vi "CheckForSaturation.vi"(8 "Replace Sat with X?":dbl=0.1 format="%#_13g", 9 "Processed Data":dbl[][](array[numeric]), 10 "Original Data In":dbl[][](array[numeric]), 11 "Bit Depth":i32=8) -> (3 "Data with Saturation":dbl[][](array[numeric]))   [LabVIEW 2022 SP3]
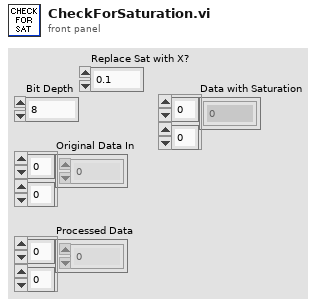
[diagram p1: front panel]
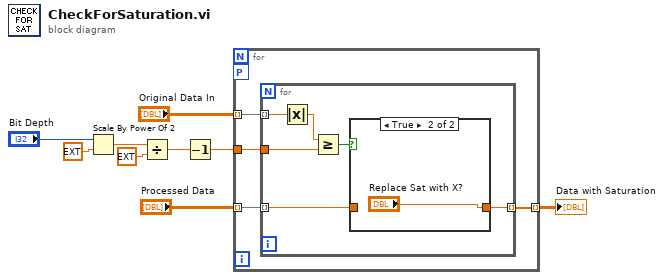
[diagram p0: block diagram]
diagram:
  n1 = Scale By Power Of 2(n="Bit Depth", x=ext 1.0) -> (x*2^n=w5:ext)
  n2 = Divide(x=w5, y=ext 2.0) -> (x/y=w7:ext)
  n3 = Decrement(x=w7) -> (x-1=w9:ext)
  n4 = for {
    tunnel: [w13] -> w2 mode=indexing
    tunnel: "Processed Data" -> [w12] mode=indexing
    workers-P: _ -> [_]
    tunnel: "Original Data In" -> [w11] mode=indexing
    tunnel: w9 -> [w10]
    n5 = for {
      tunnel: [w19] -> w13 mode=indexing
      tunnel: w12 -> [w18] mode=indexing
      tunnel: w11 -> [w17] mode=indexing
      tunnel: w10 -> [w16]
      n6 = Absolute Value(x=w17) -> (abs(x)=w14:dbl)
      n7 = Greater Or Equal?(x=w14, y=w16) -> (x >= y?=w15:bool)
      n8 = case shown="True" w15 {
        tunnel: [w20 "Replace Sat with X?"] -> w19
        tunnel: w18 -> [w20 _]
        frame False {
        }
        frame True {
        }
      }
    }
  }
  "Data with Saturation" <- w2
